vi "Write trigger.vi"(8 "error in (no error)":errorcluster, 10 "trigger":bool[][](array[boolean]), 11 "_data in":refnum<class "_data.lvclass">) -> (0 "error out":errorcluster, 3 "_data out":refnum<class "_data.lvclass">)   [LabVIEW 2019, in "_data.lvlib" / "_data.lvclass"]
uses:
  _data.lvclass
  _data.lvclass/_data.ctl
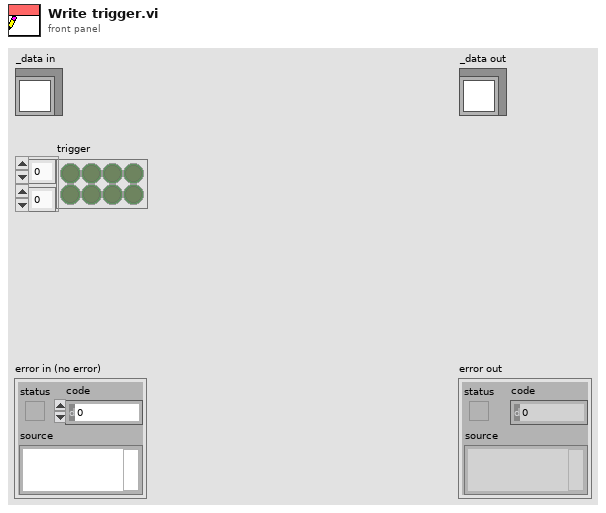
[diagram p1: front panel]
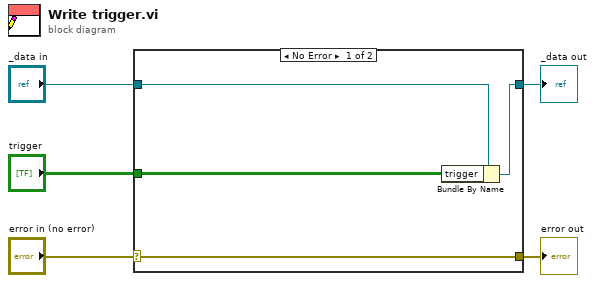
[diagram p0: block diagram]
diagram:
  n1 = case shown="No Error" "error in (no error)" {
    selector: "error in (no error)" -> [w9 w10]
    tunnel: [w9 w10] -> w4
    tunnel: [w7 w11] -> w2
    tunnel: "_data in" -> [w8 w11]
    tunnel: "trigger" -> [w6 _]
    frame No Error {
      n2 = Bundle By Name(cluster=w8, "trigger"=w6) -> (w7:refnum<class "_data.lvclass">)
    }
    frame Error {
    }
  }
  "error out" <- w4
  "_data out" <- w2
